vi "Clear ComboBox.vi"(8 "Error In":errorcluster, 11 "ComboBox Ref":refnum<vi>) -> (0 "Error Out":errorcluster)   [LabVIEW 2022 SP3]
doc: "This VI clears the contents of a ComboBox (drop-down list)."
panel:
  # "Development\nControls or indicators that are useful for development or testing, but which are not outputs of the VI."
  # "Input\nInputs to the VI"
  # "Output\nOutputs of the VI"
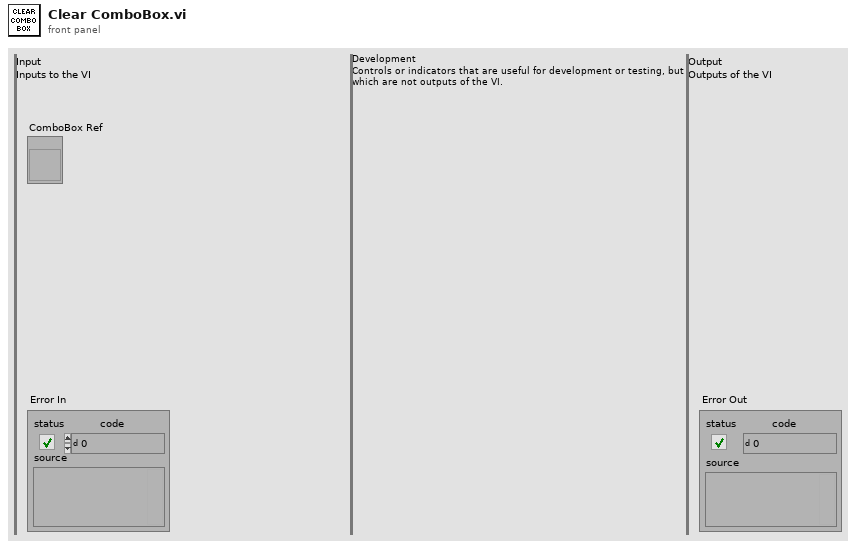
[diagram p1: front panel]
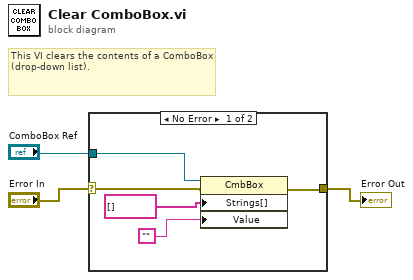
[diagram p0: block diagram]
diagram:
  # "This VI clears the contents of a ComboBox (drop-down list)."
  n1 = case shown="No Error" "Error In" {
    selector: "Error In" -> [w6 w9]
    tunnel: [w5 w9] -> w2
    tunnel: "ComboBox Ref" -> [w4 _]
    frame No Error {
      n2 = property class="CmbBox"(reference=w4, error in=w6, "Strings[]"=string[] [] ("Strings []"), "Value"="") -> (error out=w5:errorcluster)  [unwired: 1 out]
    }
    frame Error {
    }
  }
  "Error Out" <- w2
